vi "Parse input Part 2.vi"(11 "Input":string) -> (2 "Distances":u32[](array[numeric]), 3 "Times":u32[](array[numeric]))   [LabVIEW 2021]
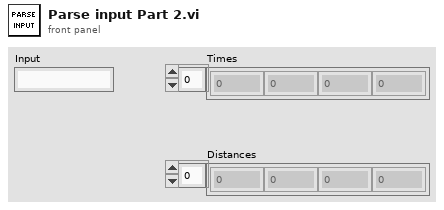
[diagram p1: front panel]
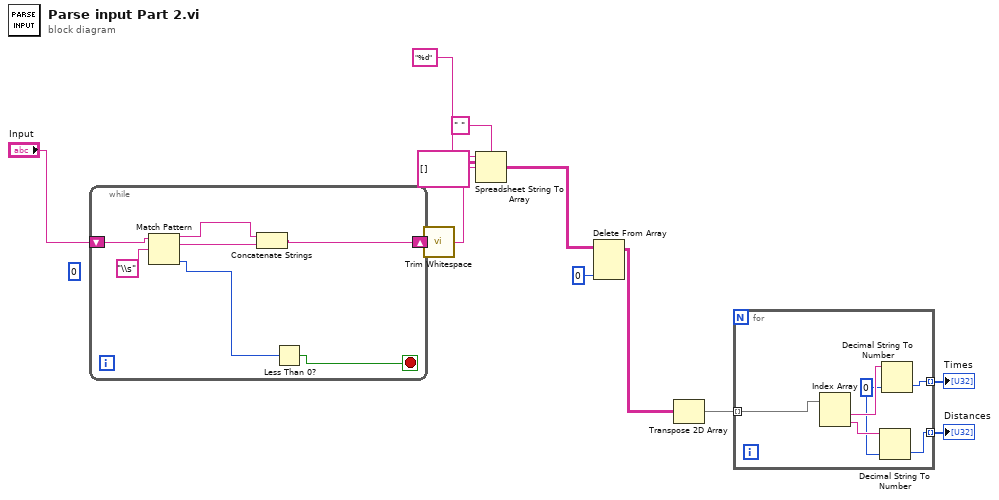
[diagram p0: block diagram]
diagram:
  (unwired) 0 ("offset past match")
  n1 = while {
    shift-right: [w15] -> w4
    shift-left: "Input" -> [w19]
    stop <- w13 stop-if-true
    n2 = Match Pattern(string=w19, regular expression="\\s") -> (before substring=w17:string, after substring=w16:string, offset past match=w14:i32)  [unwired: 1 in, 1 out]
    n3 = Concatenate Strings(w17, w16) -> (w15:string)
    n4 = Less Than 0?(x=w14) -> (x < 0?=w13:bool)
  }
  n5 = call <vilib>:"Trim Whitespace.vi"("string"=w4) -> ("trimmed string"=w12:string)  [unwired: 1 in]
  n6 = Spreadsheet String To Array(delimiter (Tab)=" ", format string="%d", spreadsheet string=w12, array type (2D Dbl)=string[][] []) -> (array=w6:string[][])
  n7 = Delete From Array(array=w6, index (col)=0 ("disabled index (col)")) -> (array with subset deleted=w8:string[][])  [unwired: 2 in, 1 out]
  n8 = Transpose 2D Array(2D array=w8) -> (transposed array=w11:string[][])
  n9 = for {
    tunnel: w11 -> [w25] mode=indexing
    tunnel: [w22] -> w10 mode=indexing
    tunnel: [w21] -> w9 mode=indexing
    w20 = u32 0 ("default (0 I32)")
    n10 = Index Array(array=w25) -> (element #1=w24:string, element #2=w23:string)  [unwired: 2 in]
    n11 = Decimal String To Number(string=w23, default (0L)=w20) -> (number=w22:u32)  [unwired: 1 in, 1 out]
    n12 = Decimal String To Number(string=w24, default (0L)=w20) -> (number=w21:u32)  [unwired: 1 in, 1 out]
  }
  "Distances" <- w10
  "Times" <- w9
